vi "test2-TestFilterJKISMStringQueueVI.vi"(8 "error in (no error)":errorcluster, 11 "TestCase in":refnum<class "testcase-CSMManagementAPI.lvclass">) -> (0 "error out":errorcluster, 3 "TestCase out":refnum<class "testcase-CSMManagementAPI.lvclass">)   [LabVIEW 2017, in "testcase-CSMManagementAPI.lvclass"]
uses:
  testcase-CSMManagementAPI.lvclass
  src/user.lib/_NEVSTOP/Communicable State Machine(CSM)/_Polymophic/CSM - Filter Interrupt Broadcasts.vi
  src/user.lib/_NEVSTOP/Communicable State Machine(CSM)/_Polymophic/CSM - Filter Status Broadcasts.vi
  src/user.lib/_NEVSTOP/Communicable State Machine(CSM)/_Polymophic/CSM - Filter Broadcasts.vi
  src/user.lib/_NEVSTOP/Communicable State Machine(CSM)/_Polymophic/CSM - Filter Sync Messages.vi
  src/user.lib/_NEVSTOP/Communicable State Machine(CSM)/_Polymophic/CSM - Filter Async without Reply Messages.vi
  src/user.lib/_NEVSTOP/Communicable State Machine(CSM)/_Polymophic/CSM - Filter Async Messages.vi
  src/user.lib/_NEVSTOP/Communicable State Machine(CSM)/_Polymophic/CSM - Filter Messges.vi
  src/user.lib/_NEVSTOP/Communicable State Machine(CSM)/_Polymophic/CSM - Filter Local States.vi
  src/user.lib/_NEVSTOP/Communicable State Machine(CSM)/_Polymophic/CSM - Filter Duplicated Lines.vi
  src/user.lib/_NEVSTOP/Communicable State Machine(CSM)/AdvanceAPI/CSM - Filter Messages to Non-Existing Modules.vi
  <vilib>/addons/_JKI Toolkits/VI Tester/TestCase.llb/TestCase.lvclass
  src/user.lib/_NEVSTOP/Communicable State Machine(CSM)/Communicable State Machine.lvlib
  C:/Program Files (x86)/National Instruments/LabVIEW 2017/vi.lib/addons/_JKI Toolkits/VI Tester/TestCase.llb/TestCase.lvclass
panel:
  out "Filter Duplicate Lines No Comments":bool
  out "Filter Duplicate Lines":bool
  out "Filter Duplicate States(Regardless of async/sync/status/interrupt)":bool
  out "Fiter Interrupt Broadcast":bool
  out "Fiter Status Broadcast":bool
  out "Fiter Broadcasts":bool
  out "Filter Messages To Non Existing CSMs":bool
  out "Filter Sync Messages":bool
  out "Filter Async Messages Without Reply":bool
  out "Filter Async Messages":bool
  out "Filter All Messages":bool
  out "Fiter Local States":bool
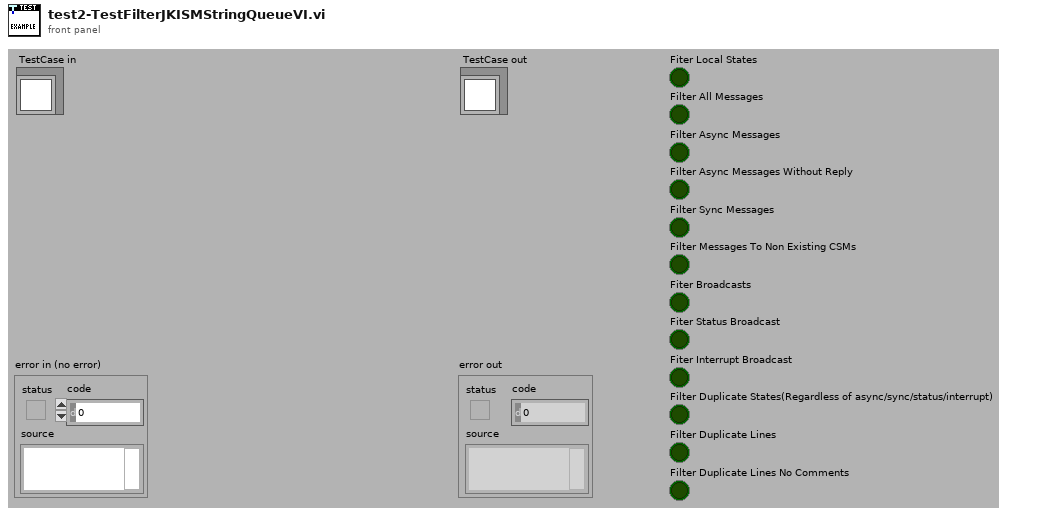
[diagram p1: front panel]
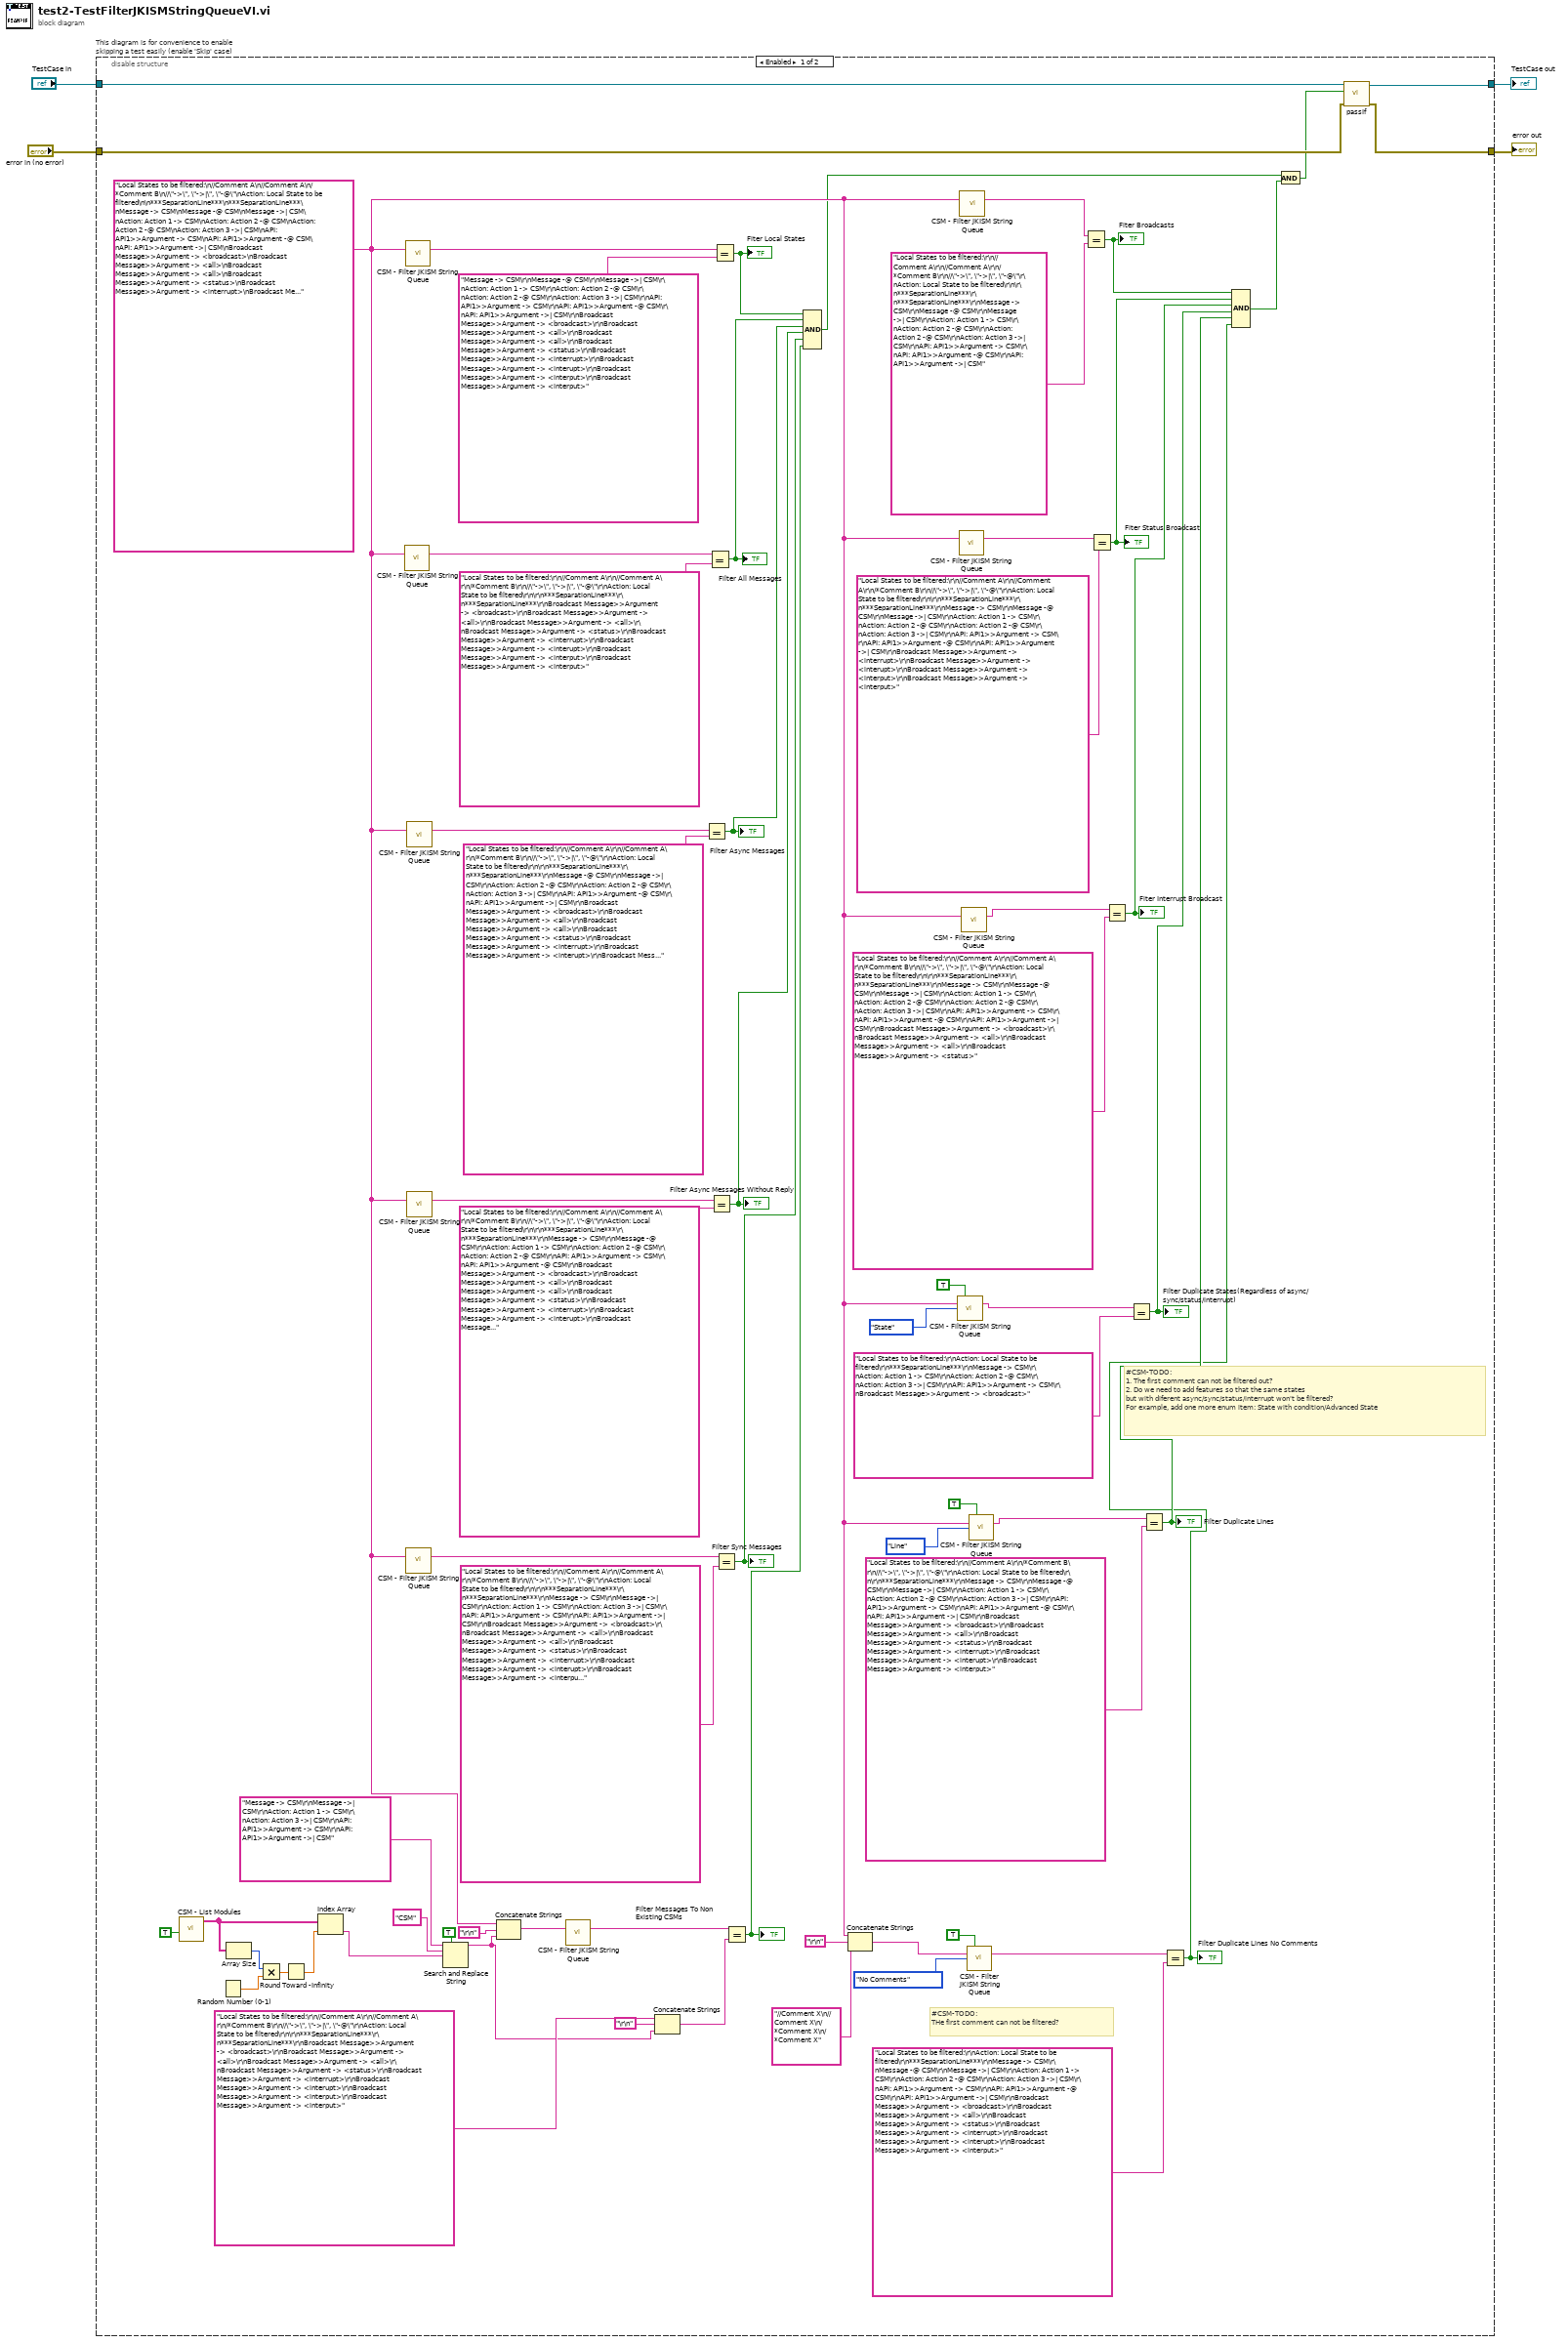
[diagram p0: block diagram]
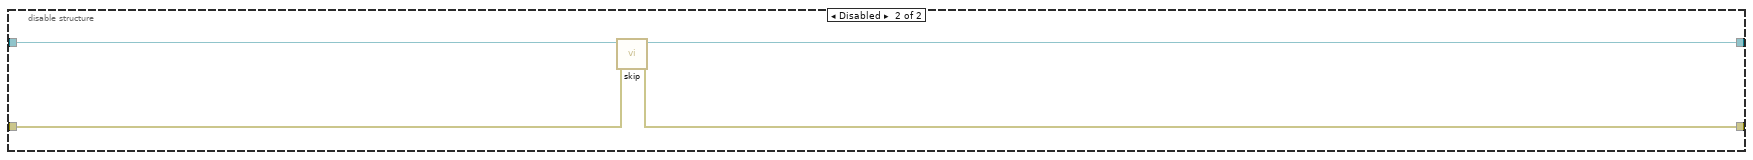
[diagram p2: hidden frame]
diagram:
  n1 = disable-structure "This diagram is for convenience to enable skipping a test easily (enable 'Skip' case)" shown="Enabled" {
    disable-tunnel: "TestCase in" -> [w25 w76]
    disable-tunnel: [w26 w74] -> w1
    disable-tunnel: [w23 w75] -> w3
    disable-tunnel: "error in (no error)" -> [w24 w73]
    frame Enabled {
      w31 = "Local States to be filtered:\n//Comment A\n//Comment A\n/*Comment B\n//\"->\", \"->|\", \"-@\"\nAction: Local State to be filtered\n\n***SeparationLine***\n***SeparationLine***\nMessage -> CSM\nMessage -@ CSM\nMessage ->| CSM\nAction: Action 1 -> CSM\nAction: Action 2 -@ CSM\nAction: Action 2 -@ CSM\nAction: Action 3 ->| CSM\nAPI: API1>>Argument -> CSM\nAPI: API1>>Argument -@ CSM\nAPI: API1>>Argument ->| CSM\nBroadcast Message>>Argument -> <broadcast>\nBroadcast Message>>Argument -> <all>\nBroadcast Message>>Argument -> <all>\nBroadcast Message>>Argument -> <status>\nBroadcast Message>>Argument -> <interrupt>\nBroadcast Message>>Argument -> <interupt>\nBroadcast Message>>Argument -> <interput>\nBroadcast Message>>Argument -> <interput>" ("States In")
      # "#CSM-TODO:\nTHe first comment can not be filtered?"
      # "#CSM-TODO:\n1. The first comment can not be filtered out?\n2. Do we need to add features so that the same states \nbut with diferent async/sync/status/interrupt won't be filtered?\nFor example, add one more enum item: State with condition/Advanced State"
      n2 = call "CSM - List Modules.vi"("With Nodes? (F)"=TRUE) -> ("Module Names"=w61:string[])  [unwired: 9 in, 1 out]
      n3 = Random Number (0-1)() -> (number: 0 to 1=w59:dbl)
      n4 = Array Size(array=w61) -> (size(s)=w60:i32)
      n5 = Multiply(x=w60, y=w59) -> (x*y=w58:dbl)
      n6 = Round Toward -Infinity(1:w58) -> (0:w57:dbl)
      n7 = Index Array(array=w61, index=w57) -> (element=w54:string)
      n8 = call-poly "CSM - Filter JKISM String Queue.vi"("States In"=w31) -> ("States Out"=w70:string)  [unwired: 14 in]
      n9 = call-poly "CSM - Filter JKISM String Queue.vi"("States In"=w31) -> ("States Out"=w72:string)  [unwired: 14 in]
      n10 = call-poly "CSM - Filter JKISM String Queue.vi"("States In"=w31) -> ("States Out"=w64:string)  [unwired: 14 in]
      n11 = call-poly "CSM - Filter JKISM String Queue.vi"("States In"=w31) -> ("States Out"=w68:string)  [unwired: 14 in]
      n12 = call-poly "CSM - Filter JKISM String Queue.vi"("States In"=w31) -> ("States Out"=w66:string)  [unwired: 14 in]
      n13 = Search and Replace String(replace all?=TRUE ("replace all? (F)"), input string="Message -> CSM\r\nMessage ->| CSM\r\nAction: Action 1 -> CSM\r\nAction: Action 3 ->| CSM\r\nAPI: API1>>Argument -> CSM\r\nAPI: API1>>Argument ->| CSM", search string="CSM", replace string=w54) -> (result string=w50:string)  [unwired: 4 in, 3 out]
      n14 = Concatenate Strings(w31, "\r\n", w50) -> (w52:string)
      n15 = call-poly "CSM - Filter JKISM String Queue.vi"("States In"=w52) -> ("States Out"=w49:string)  [unwired: 14 in]
      n16 = Concatenate Strings("Local States to be filtered:\r\n//Comment A\r\n//Comment A\r\n/*Comment B\r\n//\"->\", \"->|\", \"-@\"\r\nAction: Local State to be filtered\r\n\r\n***SeparationLine***\r\n***SeparationLine***\r\nBroadcast Message>>Argument -> <broadcast>\r\nBroadcast Message>>Argument -> <all>\r\nBroadcast Message>>Argument -> <all>\r\nBroadcast Message>>Argument -> <status>\r\nBroadcast Message>>Argument -> <interrupt>\r\nBroadcast Message>>Argument -> <interupt>\r\nBroadcast Message>>Argument -> <interput>\r\nBroadcast Message>>Argument -> <interput>" ("States Out"), "\r\n", w50) -> (w48:string)
      n17 = Equal?(x=w68, y="Local States to be filtered:\r\n//Comment A\r\n//Comment A\r\n/*Comment B\r\n//\"->\", \"->|\", \"-@\"\r\nAction: Local State to be filtered\r\n\r\n***SeparationLine***\r\n***SeparationLine***\r\nMessage -@ CSM\r\nMessage ->| CSM\r\nAction: Action 2 -@ CSM\r\nAction: Action 2 -@ CSM\r\nAction: Action 3 ->| CSM\r\nAPI: API1>>Argument -@ CSM\r\nAPI: API1>>Argument ->| CSM\r\nBroadcast Message>>Argument -> <broadcast>\r\nBroadcast Message>>Argument -> <all>\r\nBroadcast Message>>Argument -> <all>\r\nBroadcast Message>>Argument -> <status>\r\nBroadcast Message>>Argument -> <interrupt>\r\nBroadcast Message>>Argument -> <interupt>\r\nBroadcast Message>>Argument -> <interput>\r\nBroadcast Message>>Argument -> <interput>" ("States In")) -> (x = y?=w20:bool)
      "Filter Async Messages" <- w20
      n18 = Equal?(x=w70, y="Local States to be filtered:\r\n//Comment A\r\n//Comment A\r\n/*Comment B\r\n//\"->\", \"->|\", \"-@\"\r\nAction: Local State to be filtered\r\n\r\n***SeparationLine***\r\n***SeparationLine***\r\nBroadcast Message>>Argument -> <broadcast>\r\nBroadcast Message>>Argument -> <all>\r\nBroadcast Message>>Argument -> <all>\r\nBroadcast Message>>Argument -> <status>\r\nBroadcast Message>>Argument -> <interrupt>\r\nBroadcast Message>>Argument -> <interupt>\r\nBroadcast Message>>Argument -> <interput>\r\nBroadcast Message>>Argument -> <interput>" ("States In")) -> (x = y?=w21:bool)
      "Filter All Messages" <- w21
      n19 = Equal?(x=w66, y="Local States to be filtered:\r\n//Comment A\r\n//Comment A\r\n/*Comment B\r\n//\"->\", \"->|\", \"-@\"\r\nAction: Local State to be filtered\r\n\r\n***SeparationLine***\r\n***SeparationLine***\r\nMessage -> CSM\r\nMessage -@ CSM\r\nAction: Action 1 -> CSM\r\nAction: Action 2 -@ CSM\r\nAction: Action 2 -@ CSM\r\nAPI: API1>>Argument -> CSM\r\nAPI: API1>>Argument -@ CSM\r\nBroadcast Message>>Argument -> <broadcast>\r\nBroadcast Message>>Argument -> <all>\r\nBroadcast Message>>Argument -> <all>\r\nBroadcast Message>>Argument -> <status>\r\nBroadcast Message>>Argument -> <interrupt>\r\nBroadcast Message>>Argument -> <interupt>\r\nBroadcast Message>>Argument -> <interput>\r\nBroadcast Message>>Argument -> <interput>" ("States Out")) -> (x = y?=w19:bool)
      "Filter Async Messages Without Reply" <- w19
      n20 = Equal?(x=w72, y="Message -> CSM\r\nMessage -@ CSM\r\nMessage ->| CSM\r\nAction: Action 1 -> CSM\r\nAction: Action 2 -@ CSM\r\nAction: Action 2 -@ CSM\r\nAction: Action 3 ->| CSM\r\nAPI: API1>>Argument -> CSM\r\nAPI: API1>>Argument -@ CSM\r\nAPI: API1>>Argument ->| CSM\r\nBroadcast Message>>Argument -> <broadcast>\r\nBroadcast Message>>Argument -> <all>\r\nBroadcast Message>>Argument -> <all>\r\nBroadcast Message>>Argument -> <status>\r\nBroadcast Message>>Argument -> <interrupt>\r\nBroadcast Message>>Argument -> <interupt>\r\nBroadcast Message>>Argument -> <interput>\r\nBroadcast Message>>Argument -> <interput>" ("States Out")) -> (x = y?=w22:bool)
      "Fiter Local States" <- w22
      n21 = Equal?(x=w64, y="Local States to be filtered:\r\n//Comment A\r\n//Comment A\r\n/*Comment B\r\n//\"->\", \"->|\", \"-@\"\r\nAction: Local State to be filtered\r\n\r\n***SeparationLine***\r\n***SeparationLine***\r\nMessage -> CSM\r\nMessage ->| CSM\r\nAction: Action 1 -> CSM\r\nAction: Action 3 ->| CSM\r\nAPI: API1>>Argument -> CSM\r\nAPI: API1>>Argument ->| CSM\r\nBroadcast Message>>Argument -> <broadcast>\r\nBroadcast Message>>Argument -> <all>\r\nBroadcast Message>>Argument -> <all>\r\nBroadcast Message>>Argument -> <status>\r\nBroadcast Message>>Argument -> <interrupt>\r\nBroadcast Message>>Argument -> <interupt>\r\nBroadcast Message>>Argument -> <interput>\r\nBroadcast Message>>Argument -> <interput>" ("States Out")) -> (x = y?=w18:bool)
      "Filter Sync Messages" <- w18
      n22 = Equal?(x=w49, y=w48) -> (x = y?=w17:bool)
      "Filter Messages To Non Existing CSMs" <- w17
      n23 = Compound Arithmetic op=AND(w22, w21, w20, w19, w18, w17) -> (w10:bool)
      n24 = Concatenate Strings(w31, "\r\n", "//Comment X\n//Comment X\n/*Comment X\n/*Comment X" ("States Out")) -> (w28:string)
      n25 = call-poly "CSM - Filter JKISM String Queue.vi"("Keep First Matched? (T)"=TRUE, "States In"=w31, "Option"=enum16{"State", "No Comments", "Line"}."State") -> ("States Out"=w39:string)  [unwired: 12 in]
      n26 = call-poly "CSM - Filter JKISM String Queue.vi"("States In"=w31) -> ("States Out"=w45:string)  [unwired: 14 in]
      n27 = call-poly "CSM - Filter JKISM String Queue.vi"("States In"=w31) -> ("States Out"=w47:string)  [unwired: 14 in]
      n28 = call-poly "CSM - Filter JKISM String Queue.vi"("States In"=w31) -> ("States Out"=w43:string)  [unwired: 14 in]
      n29 = call-poly "CSM - Filter JKISM String Queue.vi"("Keep First Matched? (T)"=TRUE, "States In"=w28, "Option"=enum16{"State", "No Comments", "Line"}."No Comments") -> ("States Out"=w30:string)  [unwired: 12 in]
      n30 = call-poly "CSM - Filter JKISM String Queue.vi"("Keep First Matched? (T)"=TRUE, "States In"=w31, "Option"=enum16{"State", "No Comments", "Line"}."Line") -> ("States Out"=w35:string)  [unwired: 12 in]
      n31 = Equal?(x=w47, y="Local States to be filtered:\r\n//Comment A\r\n//Comment A\r\n/*Comment B\r\n//\"->\", \"->|\", \"-@\"\r\nAction: Local State to be filtered\r\n\r\n***SeparationLine***\r\n***SeparationLine***\r\nMessage -> CSM\r\nMessage -@ CSM\r\nMessage ->| CSM\r\nAction: Action 1 -> CSM\r\nAction: Action 2 -@ CSM\r\nAction: Action 2 -@ CSM\r\nAction: Action 3 ->| CSM\r\nAPI: API1>>Argument -> CSM\r\nAPI: API1>>Argument -@ CSM\r\nAPI: API1>>Argument ->| CSM" ("States Out")) -> (x = y?=w16:bool)
      "Fiter Broadcasts" <- w16
      n32 = Equal?(x=w45, y="Local States to be filtered:\r\n//Comment A\r\n//Comment A\r\n/*Comment B\r\n//\"->\", \"->|\", \"-@\"\r\nAction: Local State to be filtered\r\n\r\n***SeparationLine***\r\n***SeparationLine***\r\nMessage -> CSM\r\nMessage -@ CSM\r\nMessage ->| CSM\r\nAction: Action 1 -> CSM\r\nAction: Action 2 -@ CSM\r\nAction: Action 2 -@ CSM\r\nAction: Action 3 ->| CSM\r\nAPI: API1>>Argument -> CSM\r\nAPI: API1>>Argument -@ CSM\r\nAPI: API1>>Argument ->| CSM\r\nBroadcast Message>>Argument -> <interrupt>\r\nBroadcast Message>>Argument -> <interupt>\r\nBroadcast Message>>Argument -> <interput>\r\nBroadcast Message>>Argument -> <interput>" ("States Out")) -> (x = y?=w15:bool)
      "Fiter Status Broadcast" <- w15
      n33 = Equal?(x=w43, y="Local States to be filtered:\r\n//Comment A\r\n//Comment A\r\n/*Comment B\r\n//\"->\", \"->|\", \"-@\"\r\nAction: Local State to be filtered\r\n\r\n***SeparationLine***\r\n***SeparationLine***\r\nMessage -> CSM\r\nMessage -@ CSM\r\nMessage ->| CSM\r\nAction: Action 1 -> CSM\r\nAction: Action 2 -@ CSM\r\nAction: Action 2 -@ CSM\r\nAction: Action 3 ->| CSM\r\nAPI: API1>>Argument -> CSM\r\nAPI: API1>>Argument -@ CSM\r\nAPI: API1>>Argument ->| CSM\r\nBroadcast Message>>Argument -> <broadcast>\r\nBroadcast Message>>Argument -> <all>\r\nBroadcast Message>>Argument -> <all>\r\nBroadcast Message>>Argument -> <status>" ("States Out")) -> (x = y?=w14:bool)
      "Fiter Interrupt Broadcast" <- w14
      n34 = Equal?(x=w39, y="Local States to be filtered:\r\nAction: Local State to be filtered\r\n***SeparationLine***\r\nMessage -> CSM\r\nAction: Action 1 -> CSM\r\nAction: Action 2 -@ CSM\r\nAction: Action 3 ->| CSM\r\nAPI: API1>>Argument -> CSM\r\nBroadcast Message>>Argument -> <broadcast>" ("States Out")) -> (x = y?=w13:bool)
      "Filter Duplicate States(Regardless of async/sync/status/interrupt)" <- w13
      n35 = Equal?(x=w35, y="Local States to be filtered:\r\n//Comment A\r\n/*Comment B\r\n//\"->\", \"->|\", \"-@\"\r\nAction: Local State to be filtered\r\n\r\n***SeparationLine***\r\nMessage -> CSM\r\nMessage -@ CSM\r\nMessage ->| CSM\r\nAction: Action 1 -> CSM\r\nAction: Action 2 -@ CSM\r\nAction: Action 3 ->| CSM\r\nAPI: API1>>Argument -> CSM\r\nAPI: API1>>Argument -@ CSM\r\nAPI: API1>>Argument ->| CSM\r\nBroadcast Message>>Argument -> <broadcast>\r\nBroadcast Message>>Argument -> <all>\r\nBroadcast Message>>Argument -> <status>\r\nBroadcast Message>>Argument -> <interrupt>\r\nBroadcast Message>>Argument -> <interupt>\r\nBroadcast Message>>Argument -> <interput>" ("States Out")) -> (x = y?=w12:bool)
      "Filter Duplicate Lines" <- w12
      n36 = Equal?(x=w30, y="Local States to be filtered:\r\nAction: Local State to be filtered\r\n***SeparationLine***\r\nMessage -> CSM\r\nMessage -@ CSM\r\nMessage ->| CSM\r\nAction: Action 1 -> CSM\r\nAction: Action 2 -@ CSM\r\nAction: Action 3 ->| CSM\r\nAPI: API1>>Argument -> CSM\r\nAPI: API1>>Argument -@ CSM\r\nAPI: API1>>Argument ->| CSM\r\nBroadcast Message>>Argument -> <broadcast>\r\nBroadcast Message>>Argument -> <all>\r\nBroadcast Message>>Argument -> <status>\r\nBroadcast Message>>Argument -> <interrupt>\r\nBroadcast Message>>Argument -> <interupt>\r\nBroadcast Message>>Argument -> <interput>" ("States Out")) -> (x = y?=w11:bool)
      "Filter Duplicate Lines No Comments" <- w11
      n37 = Compound Arithmetic op=AND(w16, w15, w14, w13, w12, w11) -> (w9:bool)
      n38 = And(x=w10, y=w9) -> (x .and. y?=w8:bool)
      n39 = call-dynamic "passIf.vi"("error in (no error)"=w24, "pass"=w8, "TestCase in"=w25) -> ("error out"=w23:errorcluster, "TestCase out"=w26:refnum<class "testcase-CSMManagementAPI.lvclass">)  [unwired: 7 in]
    }
    frame Disabled {
      # "skip test result while test is under development"
      n40 = call <vilib>:"skip.vi"("error in (no error)"=w73, "TestCase in"=w76) -> ("error out"=w75:errorcluster, "TestCase out"=w74:refnum<class "testcase-CSMManagementAPI.lvclass">)  [unwired: 8 in]
    }
  }
  "error out" <- w3
  "TestCase out" <- w1
